vi "Find FPGA Target.vi"(8 "error in (no error)":errorcluster, 10 "FPGA Target Name":string, 11 "Project in":refnum<vi>) -> (0 "error out":errorcluster, 2 "TargetItem out":refnum<vi>, 3 "Project out":refnum<vi>)   [LabVIEW 2015, in "Project.lvclass"]
uses:
  Project.lvclass
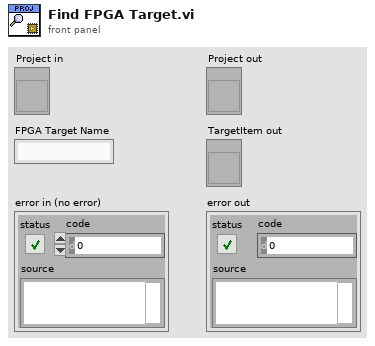
[diagram p1: front panel]
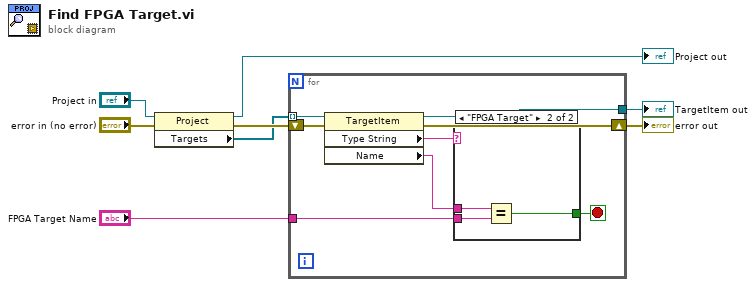
[diagram p0: block diagram]
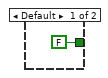
[diagram p2: hidden frame]
diagram:
  n1 = property class="Project"(reference="Project in", error in="error in (no error)") -> (reference out=→"Project out":refnum<vi>, error out=w3:errorcluster, "Targets"=w2:refnum<vi>[])
  n2 = for {
    tunnel: w2 -> [w16] mode=indexing
    tunnel: "FPGA Target Name" -> [w15]
    shift-right: [w12] -> w4
    shift-left: w3 -> [w13]
    tunnel: [w11] -> w5
    stop <- w10 stop-if-true
    n3 = property class="TargetItem"(reference=w16, error in=w13) -> (reference out=w11:refnum<vi>, error out=w12:errorcluster, "Type String"=w9:string, "Name"=w14:string)
    n4 = case shown="\"FPGA Target\"" w9 {
      tunnel: w15 -> [_ w20]
      tunnel: w14 -> [_ w19]
      tunnel: [FALSE w18] -> w10
      frame Default {
      }
      frame "FPGA Target" {
        n5 = Equal?(x=w19, y=w20) -> (x = y?=w18:bool)
      }
    }
  }
  "TargetItem out" <- w5
  "error out" <- w4
